vi "Voltage_to_unsigned_16bit_3(SubVI).vi"(11 "Voltage_in":dbl) -> (3 "unsigned 16bit integer":u16)   [LabVIEW 2016]
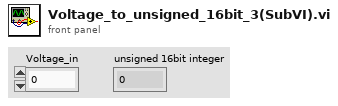
[diagram p1: front panel]
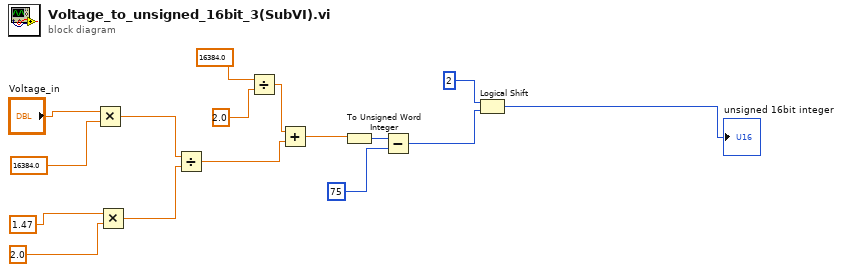
[diagram p0: block diagram]
diagram:
  n1 = Multiply(x="Voltage_in", y=16384.0) -> (x*y=w10:dbl)
  n2 = Multiply(x=1.47, y=2.0) -> (x*y=w11:dbl)
  n3 = Divide(x=w10, y=w11) -> (x/y=w15:dbl)
  n4 = Divide(x=16384.0, y=2.0) -> (x/y=w14:dbl)
  n5 = Add(x=w14, y=w15) -> (x+y=w16:dbl)
  n6 = To Unsigned Word Integer(number=w16) -> (unsigned 16bit integer=w3:u16)
  n7 = Subtract(x=w3, y=u16 75) -> (x-y=w2:u16)
  n8 = Logical Shift(y=2, x=w2) -> (x << y=→"unsigned 16bit integer":u16)
